vi "Investigate SCTL Errors.vi"() -> ()   [LabVIEW 2010]
uses:
  <vilib>/eio/EIONode/EIONode.xnode
  <vilib>/rvi/eio/nirviEIOImplementation/nirviEIOImplementation.xnode
  <vilib>/rvi/eio/common/nirviEmuClasses.ctl
  <vilib>/Platform/TimedLoop/XDataNode/XDataNode.xnode
  <vilib>/Platform/TimedLoop/XDataNode/timing_clust.ctl
  <vilib>/Platform/TimedLoop/XDataNode/nitl_modes.ctl
  <vilib>/Platform/TimedLoop/XDataNode/wakeup.ctl
  <vilib>/rvi/eio/common/nirviEmuTemplateMethod_noerrors.vi
  <vilib>/Platform/TimedLoop/XDataNode/XDNodeRunTimeDep.lvlib
panel:
  in  "stop":bool
  out "Average Acceleration":fxp<+/-,26,6> format="%.35g"
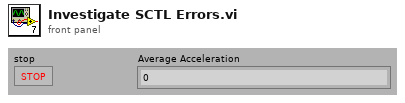
[diagram p1: front panel]
types:
  T1 = typedef "nirviEmuClasses.ctl" = enum16{"IO Read", "IO Write", "Method", "Property Read", "Property Write"}
  T2 = typedef "XDNodeRunTimeDep.lvlib/timing_clust.ctl" = cluster{"Expected End [f-1]":u64, "Actual End [f-1]":u64, "Finished Late? [f-1]":bool, "Expected End [i-1]":u64, "Actual End [i-1]":u64, "Finished Late? [i-1]":bool, "Expected Start [i]":u64, "Actual Start [i]":u64, "Expected Start [f]":u64, "Actual Start [f]":u64, "Source Name":string, "Structure Name":string, "Period":i64, "Deadline":i64, "Offset":i64, "Start":i64, "Priority":i32, "Timeout":i32, "Mode":T3, "Wakeup Reason":T4, "Error":errorcluster, "Source Type":string, "Secondary Source Type":string, "Global End Time":u64, "Global Start Time":u64, "Frame Duration":u64, "Iteration Duration":u64, "Assigned CPU":i32, "I/O Scan Engine Mode":u32}
  T3 = typedef "XDNodeRunTimeDep.lvlib/nitl_modes.ctl" = enum32{"No Change", "Process missed periods, maintain original phase", "Discard missed periods, maintain original phase", "Process missed periods, ignore original phase", "Discard missed periods, ignore original phase"}
  T4 = typedef "XDNodeRunTimeDep.lvlib/wakeup.ctl" = enum32{"Normal", "Aborted", "Asynchronous wakeup", "Timing source error", "Timed loop error", "Timeout"}
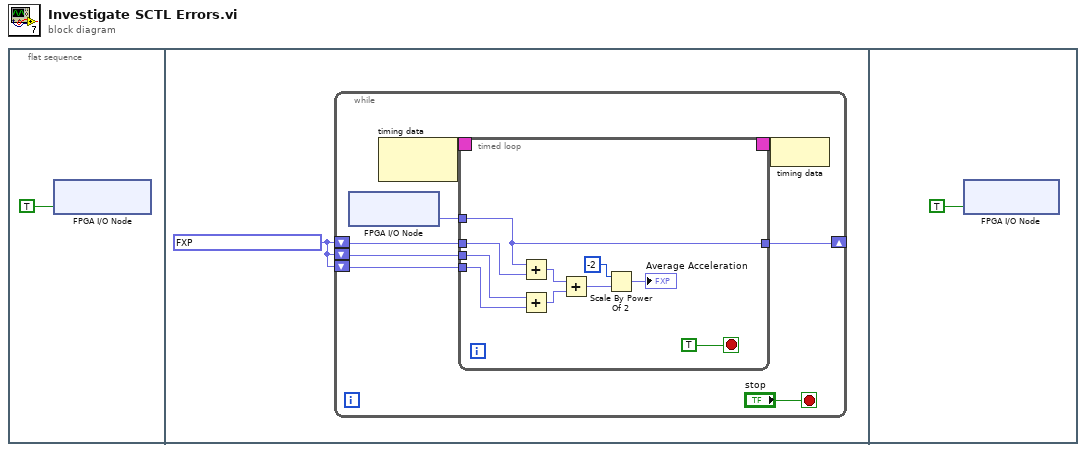
[diagram p0: block diagram]
diagram:
  n1 = flat-sequence {
    frame #0 {
      n2 = xnode "FPGA I/O Node"("Mod2/Start"=TRUE) -> ()  [unwired: 1 in, 1 out]
    }
    frame #1 {
      w13 = fxp<+/-,24,4> 0.0 ("Mod2/AI0")
      n3 = while {
        shift-right: [w14] -> _
        shift-left: w13 -> [w17]
        shift-left: w13 -> [w16]
        shift-left: w13 -> [w15]
        stop <- "stop" stop-if-true
        n4 = xnode "FPGA I/O Node"() -> ("Mod2/AI0"=w19:fxp<+/-,24,4>)  [unwired: 1 in, 1 out]
        n5 = node-c288() -> (w21:T2)  [unwired: 1 in]
        n6 = timed-loop {
          timing: w21 -> [_]
          timing-out: [_] -> w20
          tunnel: w19 -> [w41]
          tunnel: w17 -> [w44]
          tunnel: w16 -> [w43]
          tunnel: w15 -> [w42]
          tunnel: [w41] -> w14
          stop <- TRUE stop-if-true
          n7 = Add(x=w41, y=w44) -> (x+y=w50:fxp<+/-,25,5>)
          n8 = Add(x=w43, y=w42) -> (x+y=w49:fxp<+/-,25,5>)
          n9 = Add(x=w50, y=w49) -> (x+y=w47:fxp<+/-,26,6>)
          n10 = Scale By Power Of 2(n=-2, x=w47) -> (x*2^n=→"Average Acceleration":fxp<+/-,26,6>)
        }
        n11 = node-c288(w20) -> ()
      }
    }
    frame #2 {
      n12 = xnode "FPGA I/O Node"("Mod2/Stop"=TRUE) -> ()  [unwired: 1 in, 1 out]
    }
  }
